vi "Repeat_Program_Prompt.vi"(8 "error in (no error)":errorcluster) -> (0 "error out":errorcluster, 3 "Yes":bool)   [LabVIEW 2018]
doc: "This VI prompts the user to choose whether to run another test or to terminate the program.\n\nInputs:\nError in.\n\nOutputs:\nError out;\nYes."
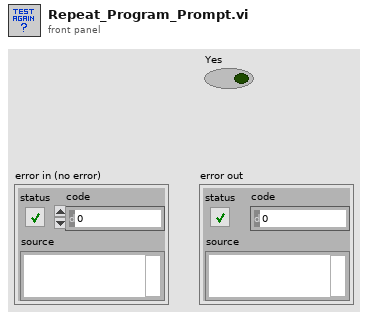
[diagram p1: front panel]
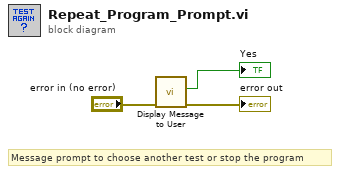
[diagram p0: block diagram]
diagram:
  # "Message prompt to choose another test or stop the program"
  n1 = call "Display Message to User"("error in (no error)"="error in (no error)") -> ("error out"=→"error out":errorcluster, "Yes"=→"Yes":bool)  [unwired: 9 in]
